vi "mono_simulator_config.vi"() -> ()   [LabVIEW 2018]
uses:
  Simulator_Configuration.ctl
panel:
  in  "?":T1
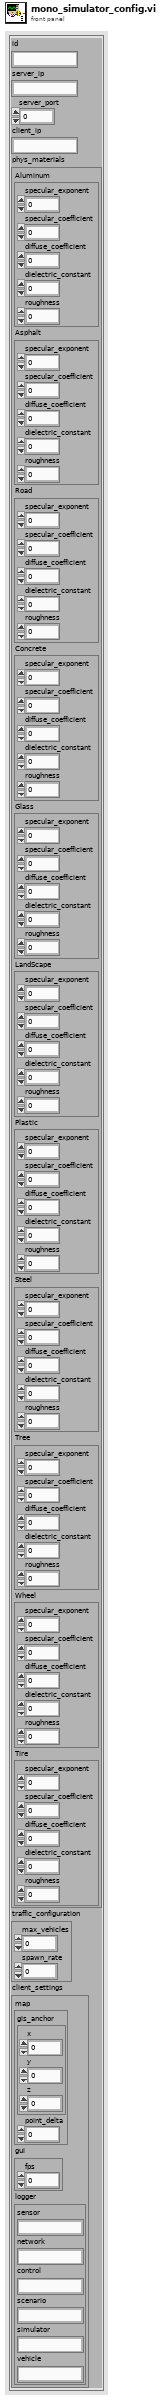
[diagram p1: front panel]
types:
  T1 = typedef "Simulator_Configuration.ctl" = cluster{"id":string, "server_ip":string, "server_port":i32, "client_ip":string, "phys_materials":cluster{"Aluminum":cluster{"specular_exponent":i32, "specular_coefficient":i32, "diffuse_coefficient":i32, "dielectric_constant":i32, "roughness":i32}, "Asphalt":cluster{"specular_exponent":i32, "specular_coefficient":i32, "diffuse_coefficient":i32, "dielectric_constant":i32, "roughness":i32}, "Road":cluster{"specular_exponent":i32, "specular_coefficient":i32, "diffuse_coefficient":i32, "dielectric_constant":i32, "roughness":i32}, "Concrete":cluster{"specular_exponent":i32, "specular_coefficient":i32, "diffuse_coefficient":i32, "dielectric_constant":i32, "roughness":i32}, "Glass":cluster{"specular_exponent":i32, "specular_coefficient":i32, "diffuse_coefficient":i32, "dielectric_constant":i32, "roughness":i32}, "LandScape":cluster{"specular_exponent":i32, "specular_coefficient":i32, "diffuse_coefficient":i32, "dielectric_constant":i32, "roughness":i32}, "Plastic":cluster{"specular_exponent":i32, "specular_coefficient":i32, "diffuse_coefficient":i32, "dielectric_constant":i32, "roughness":i32}, "Steel":cluster{"specular_exponent":i32, "specular_coefficient":i32, "diffuse_coefficient":i32, "dielectric_constant":i32, "roughness":i32}, "Tree":cluster{"specular_exponent":i32, "specular_coefficient":i32, "diffuse_coefficient":i32, "dielectric_constant":i32, "roughness":i32}, "Wheel":cluster{"specular_exponent":i32, "specular_coefficient":i32, "diffuse_coefficient":i32, "dielectric_constant":i32, "roughness":i32}, "Tire":cluster{"specular_exponent":i32, "specular_coefficient":i32, "diffuse_coefficient":i32, "dielectric_constant":i32, "roughness":i32}}, "traffic_configuration":cluster{"max_vehicles":i32, "spawn_rate":i32}, "client_settings":cluster{"map":cluster{"gis_anchor":cluster{"x":i32, "y":i32, "z":i32}, "point_delta":i32}, "gui":cluster{"fps":i32}, "logger":cluster{"sensor":string, "network":string, "control":string, "scenario":string, "simulator":string, "vehicle":string}}}
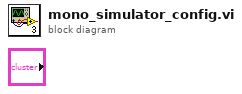
[diagram p0: block diagram]
diagram:
